vi "Set Stream Reader.vi"(4 "ms timeout (-1)":i32=-1, 7 "StreamReader":refnum<vi>, 8 "error in":errorcluster, 10 "UserData":variant, 11 "GLue in":refnum<class "class.GLue.lvclass">) -> (0 "error out":errorcluster, 3 "GLue out":refnum<class "class.GLue.lvclass">)   [LabVIEW 2014, in "GLue.lvlib"]
doc: "Adds a GLue module with the provided name to the GLue instance.\n\n<B>Parameter(s) </B>\n-----------------\n\n- <B>GLue in:</B> Reference to the GLue instance.\n\n- <B>GLue Module:</B> A LabVIEW VI reference to a GLue module which exposes LabVIEW code to Lua.\n\n- <B>User Data:</B> User supplied data that will be made available when the module is invoked.\n\n- <B>ms timeout (-1):</B> The time to wait for the GLue reference to become available. A value of '-1' specifies an infinite timeout.\n\n- <B>error in:</B> Describes error conditions that occur before this VI runs. This input provides standard error in functionality. \n\n- <B>GLue out:</B> Reference to the GLue instance.\n\n- <B>error out:</B> Contains error information. This output provides standard error out functionality."
uses:
  GLue.lvlib
  Private/Class/class.GLue.lvclass
panel:
  # "Input"
  # "Output"
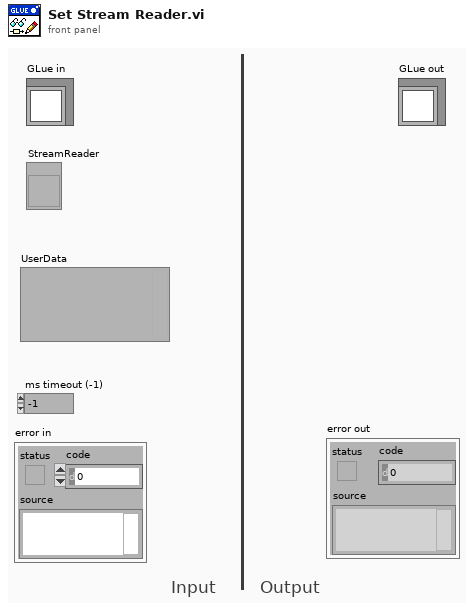
[diagram p1: front panel]
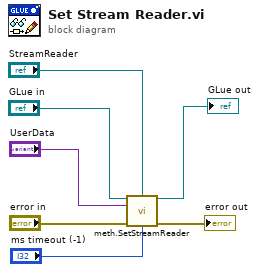
[diagram p0: block diagram]
diagram:
  n1 = call "meth.SetStreamReader.vi"("class.GLue in"="GLue in", "StreamReader"="StreamReader", "UserData"="UserData", "error in"="error in", "ms timeout (-1)"="ms timeout (-1)") -> ("class.GLue out"=→"GLue out":refnum<class "class.GLue.lvclass">, "error out"=→"error out":errorcluster)  [unwired: 9 in]
